vi "Test Cage Diagram API.vi"() -> ()   [LabVIEW 2018]
doc: "Cage Diagram API Tester."
uses:
  Typedefs/CTL_Cage_type.ctl
  <vilib>/Utility/miscctls.llb/LVPointTypeDef.ctl
  Cage Diagram.lvlib
panel:
  in  "Test param 2":string="dtyjusdtyjdty"
  in  "Test param 1":dbl=17.0
  in  "Cage type":T1 items=["Round", "Square", "Donut maze", "T-maze", "Sociability maze", ""]
  in  "New Layout":bool
  in  "Show Block Diagram":bool
  in  "Stop Module":bool
  in  "Start Module":bool
  in  "Hide Module Panel":bool
  in  "Show Module Panel":bool
  out "Status":string
  out "Module Running?":bool
  # "This VI tests the API for the Module."
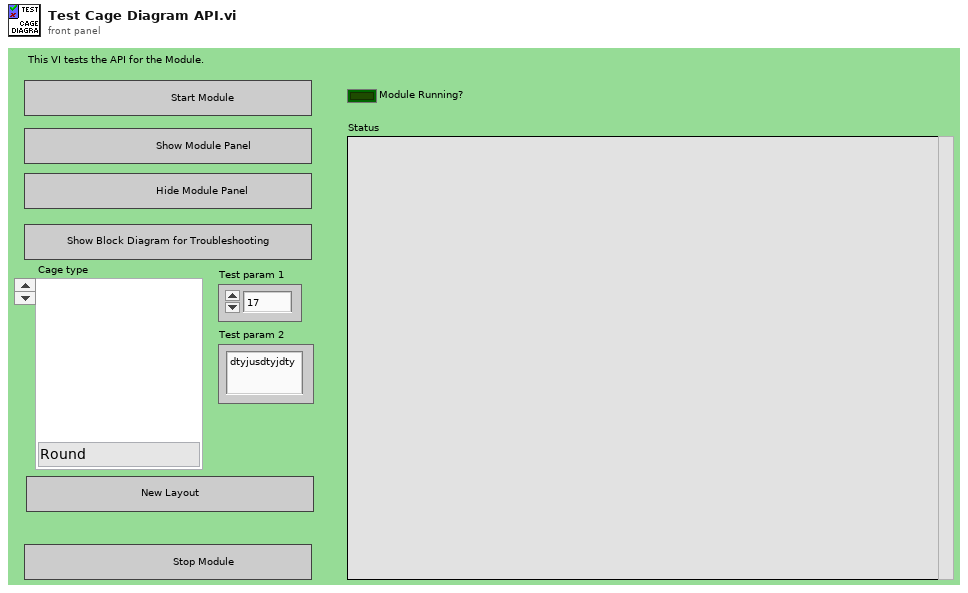
[diagram p1: front panel]
types:
  T1 = typedef "Cage Diagram.lvlib/CTL_Cage_type.ctl" = u16
  T2 = typedef "LVPointTypeDef.ctl" = cluster{"Horizontal":i16, "Vertical":i16}
  T3 = typedef "Cage Diagram.lvlib/Broadcast Events--cluster.ctl" = cluster{"Module Did Init":refnum<user-event>, "Status Updated":refnum<user-event>, "Error Reported":refnum<user-event>, "Module Did Stop":refnum<user-event>, "Update Module Execution Status":refnum<user-event>, "Broadcast New Layout":refnum<user-event>}
  T4 = cluster{"Test param 1":dbl, "Test param 2":string}
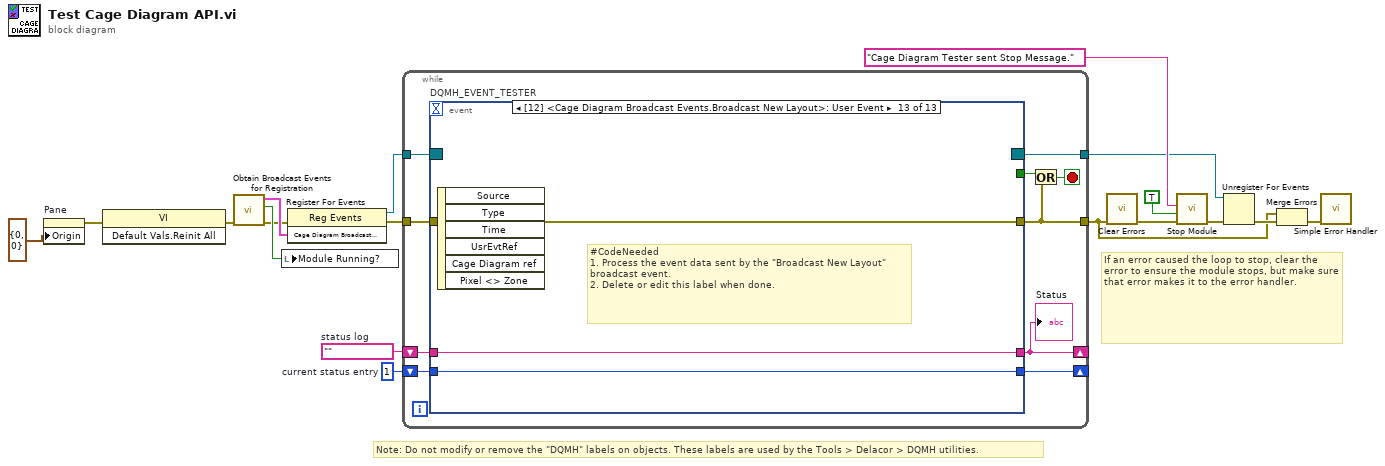
[diagram p0: block diagram]
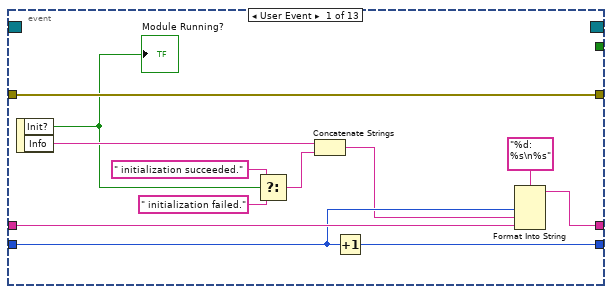
[diagram p2: hidden frame]
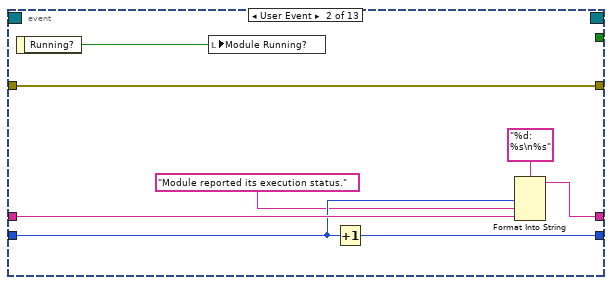
[diagram p3: hidden frame]
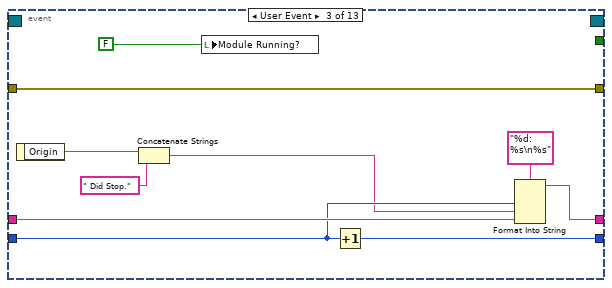
[diagram p4: hidden frame]
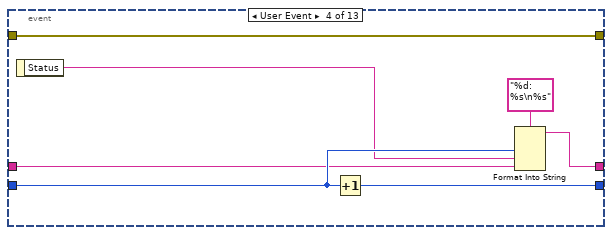
[diagram p5: hidden frame]
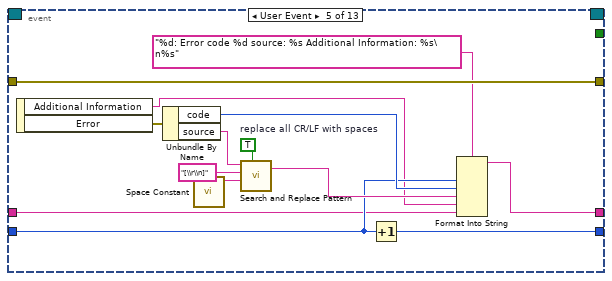
[diagram p6: hidden frame]
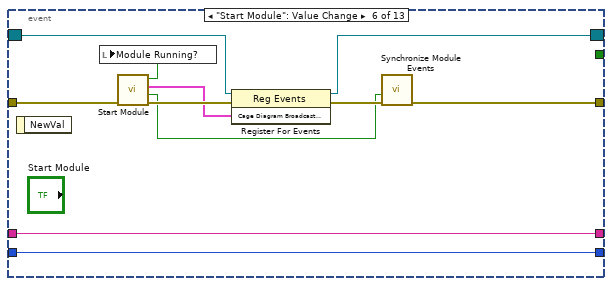
[diagram p7: hidden frame]
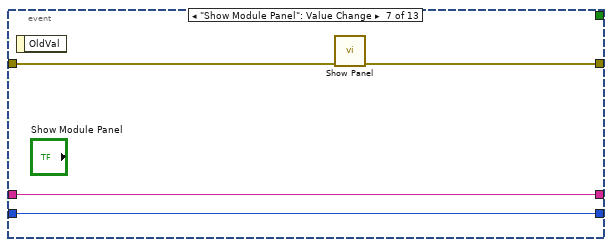
[diagram p8: hidden frame]
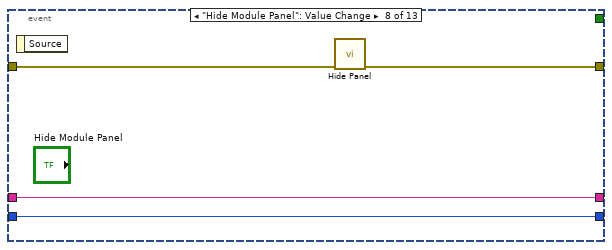
[diagram p9: hidden frame]
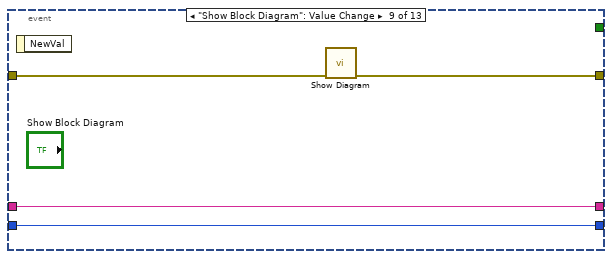
[diagram p10: hidden frame]
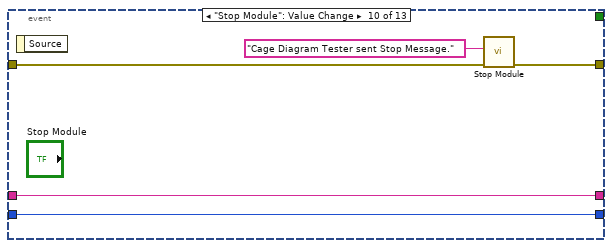
[diagram p11: hidden frame]
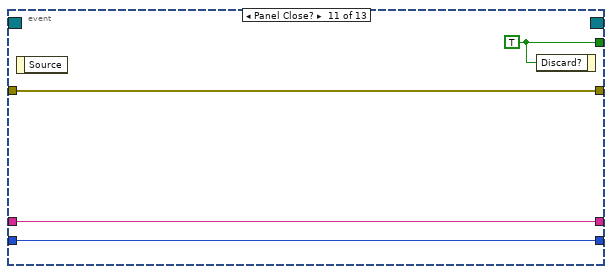
[diagram p12: hidden frame]
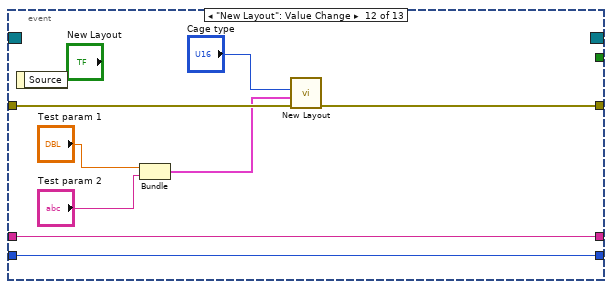
[diagram p13: hidden frame]
diagram:
  w14 = 1  # current status entry
  w15 = ""  # status log
  # "If an error caused the loop to stop, clear the error to ensure the module stops, but make sure that error makes it to the error handler."
  # "Note: Do not modify or remove the \"DQMH\" labels on objects. These labels are used by the Tools > Delacor > DQMH utilities."
  n1 = property on="Pane" class="Pane"("Origin"=T2 {"Horizontal"=0, "Vertical"=0}) -> (error out=w1:errorcluster)  [unwired: 2 in, 1 out]
  n2 = invoke class="VI" method="Default Vals.Reinit All"(error in=w1) -> (error out=w4:errorcluster)  [unwired: 2 in, 2 out]
  n3 = call "Obtain Broadcast Events for Registration.vi"("error in (no error)"=w4) -> ("error out"=w3:errorcluster, "Already running?"=w5:bool, "Cage Diagram Broadcast Events"=w12:T3)  [unwired: 8 in]
  n4 = local write "Module Running?"(w5) -> ()
  n5 = register-events(error in=w3, w12) -> (reference out=w11:refnum<event-registration>, error out=w13:errorcluster)  [unwired: 1 in]
  n6 = while {
    tunnel: w11 -> [w28]
    tunnel: [w19] -> w6
    shift-right: [w23] -> _
    shift-left: w15 -> [w25]
    shift-right: [w24] -> _
    shift-left: w14 -> [w26]
    tunnel: w13 -> [w21]
    tunnel: [w20] -> w10
    stop <- w22 stop-if-true
    n7 = event "DQMH_EVENT_TESTER" shown="[12] <Cage Diagram Broadcast Events.Broadcast New Layout>: User Event" {
      selector: w28 -> [_ _ _ _ _ w84 _ _ _ _ _ _ _]
      dyn-events: [_ _ _ _ _ w83 _ _ _ _ _ _ _] -> w20
      timeout: _ -> [_ _ _ _ _ _ _ _ _ _ _ _ _]
      tunnel: [_ _ _ _ _ _ _ _ _ _ w111 _ _] -> w27
      tunnel: [w40 w42 w49 w59 w79 w82 w94 w98 w99 w105 w108 w116 w122] -> w19
      tunnel: w26 -> [w37 w46 w56 w62 w69 w87 w92 w96 w100 w106 w109 w117 w120]
      tunnel: w25 -> [w38 w47 w57 w61 w67 w88 w93 w97 w101 w107 w110 w118 w121]
      tunnel: [w35 w44 w54 w63 w70 w88 w93 w97 w101 w107 w110 w118 w121] -> w23
      tunnel: [w36 w45 w55 w65 w68 w87 w92 w96 w100 w106 w109 w117 w120] -> w24
      tunnel: w21 -> [w40 w42 w49 w59 w79 w81 w91 w95 w102 w103 w108 w119 w122]
      event User Event {
        n8 = event-data() -> ("Init?"=w32:bool, "Info"=w34:string)  [unwired: 1 in]
        "Module Running?" <- w32
        n9 = Select(t=" initialization succeeded.", s=w32, f=" initialization failed.") -> (s? t:f=w29:string)
        n10 = Concatenate Strings(w34, w29) -> (w33:string)
        n11 = Increment(x=w37) -> (x+1=w36:i32)
        n12 = Format Into String(format string="%d: %s\n%s", w37, w33, w38) -> (resulting string=w35:string)  [unwired: 2 in, 1 out]
      }
      event User Event {
        n13 = event-data() -> ("Running?"=w41:bool)  [unwired: 1 in]
        n14 = local write "Module Running?"(w41) -> ()
        n15 = Increment(x=w46) -> (x+1=w45:i32)
        n16 = Format Into String(format string="%d: %s\n%s", w46, "Module reported its execution status.", w47) -> (resulting string=w44:string)  [unwired: 2 in, 1 out]
      }
      event User Event {
        n17 = event-data() -> ("Origin"=w53:string)  [unwired: 1 in]
        n18 = Concatenate Strings(w53, " Did Stop.") -> (w52:string)
        n19 = local write "Module Running?"(FALSE ("Module Did Init?")) -> ()
        n20 = Increment(x=w56) -> (x+1=w55:i32)
        n21 = Format Into String(format string="%d: %s\n%s", w56, w52, w57) -> (resulting string=w54:string)  [unwired: 2 in, 1 out]
      }
      event User Event {
        n22 = event-data() -> ("Status"=w60:string)  [unwired: 1 in]
        n23 = Increment(x=w62) -> (x+1=w65:i32)
        n24 = Format Into String(format string="%d: %s\n%s", w62, w60, w61) -> (resulting string=w63:string)  [unwired: 2 in, 1 out]
      }
      event User Event {
        w75 = TRUE  # replace all CR/LF with spaces
        n25 = event-data() -> ("Additional Information"=w66:string, "Error"=w71:errorcluster)  [unwired: 1 in]
        n26 = Unbundle By Name(w71) -> ("code"=w72:i32, "source"=w73:string)
        n27 = call <vilib>:"Space Constant.vi"() -> ("String"=w76:string)
        n28 = call <vilib>:"Search and Replace Pattern.vi"("string"=w73, "regular expression (\"\")"="[\\r\\n]" ("regular expression (\"\")"), "replace string (\"\")"=w76, "replace all? (F)"=w75) -> ("result string"=w74:string)  [unwired: 1 in, 1 out]
        n29 = Increment(x=w69) -> (x+1=w68:i32)
        n30 = Format Into String(format string="%d: Error code %d source: %s Additional Information: %s\n%s", w69, w72, w74, w66, w67) -> (resulting string=w70:string)  [unwired: 2 in, 1 out]
      }
      event "Start Module": Value Change {
        n31 = event-data() -> ()  [unwired: 1 in, 1 out]
        n32 = call "Start Module.vi"("error in (no error)"=w81) -> ("error out"=w89:errorcluster, "Wait for Event Sync?"=w86:bool, "Cage Diagram Broadcast Events"=w85:T3, "Module Was Already Running?"=w80:bool)  [unwired: 7 in]
        n33 = local write "Module Running?"(w80) -> ()
        n34 = register-events(reference=w84, error in=w89, w85) -> (reference out=w83:refnum<event-registration>, error out=w90:errorcluster)
        n35 = call "Synchronize Module Events.vi"("error in (no error)"=w90, "Wait for Event Sync?"=w86) -> ("error out"=w82:errorcluster)  [unwired: 9 in]
      }
      event "Show Module Panel": Value Change {
        n36 = event-data() -> ()  [unwired: 1 in, 1 out]
        n37 = call "Show Panel.vi"("error in (no error)"=w91) -> ("error out"=w94:errorcluster)  [unwired: 10 in]
      }
      event "Hide Module Panel": Value Change {
        n38 = event-data() -> ()  [unwired: 1 in, 1 out]
        n39 = call "Hide Panel.vi"("error in (no error)"=w95) -> ("error out"=w98:errorcluster)  [unwired: 10 in]
      }
      event "Show Block Diagram": Value Change {
        n40 = event-data() -> ()  [unwired: 1 in, 1 out]
        n41 = call "Show Diagram.vi"("error in (no error)"=w102) -> ("error out"=w99:errorcluster)  [unwired: 10 in]
      }
      event "Stop Module": Value Change {
        n42 = event-data() -> ()  [unwired: 1 in, 1 out]
        n43 = call "Stop Module.vi"("error in (no error)"=w103, "Origin"="Cage Diagram Tester sent Stop Message.") -> ("error out"=w105:errorcluster)  [unwired: 9 in]
      }
      event Panel Close? {
        w111 = TRUE ("Discard?")
        n44 = event-data() -> ()  [unwired: 1 in, 1 out]
        n45 = event-data("Discard?"=w111) -> ()  [unwired: 1 in, 1 out]
      }
      event "New Layout": Value Change {
        n46 = event-data() -> ()  [unwired: 1 in, 1 out]
        n47 = Bundle("Test param 1"="Test param 1", "Test param 2"="Test param 2") -> (w112:T4)  [unwired: 1 in]
        n48 = call "New Layout.vi"("error in (no error)"=w119, "Cage parameters"=w112, "Cage type"="Cage type") -> ("error out"=w116:errorcluster)  [unwired: 8 in]
      }
      event User Event {
        # "#CodeNeeded\n1. Process the event data sent by the \"Broadcast New Layout\" broadcast event.\n2. Delete or edit this label when done."
        n49 = event-data() -> ()  [unwired: 1 in, 6 out]
      }
    }
    "Status" <- w23
    n50 = Or(x=w27, y=w19) -> (x .or. y?=w22:bool)
  }
  n51 = call <vilib>:"Clear Errors.vi"("error in (no error)"=w6) -> ("error out"=w8:errorcluster)  [unwired: 5 in, 1 out]
  n52 = call "Stop Module.vi"("error in (no error)"=w8, "Wait for Module to Stop? (F)"=TRUE ("Wait for Module to stop?"), "Origin"="Cage Diagram Tester sent Stop Message.") -> ("error out"=w17:errorcluster)  [unwired: 8 in]
  n53 = Unregister For Events(event registration refnum=w10, error in=w17) -> (error out=w18:errorcluster)
  n54 = Merge Errors(w6, w18) -> (w7:errorcluster)
  n55 = call <vilib>:"Simple Error Handler.vi"("error in (no error)"=w7) -> ()  [unwired: 4 in, 5 out]
